vi "Globals.vi"() -> ()   [LabVIEW 2013]
panel:
  out "slide":dbl
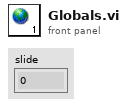
[diagram p1: front panel]
diagram:
